vi "Populate Font Control.vi"(8 "error in (no error)":errorcluster, 10 "Font in":string, 11 "DNL_Font":refnum<vi>) -> (0 "error out":errorcluster, 2 "Font out":string)   [LabVIEW 2012]
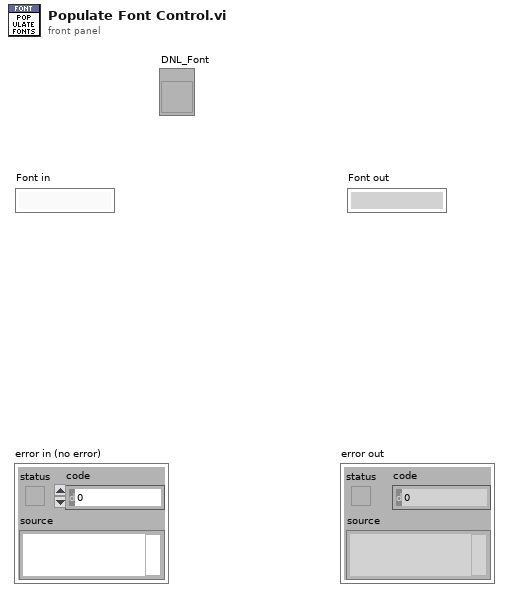
[diagram p1: front panel]
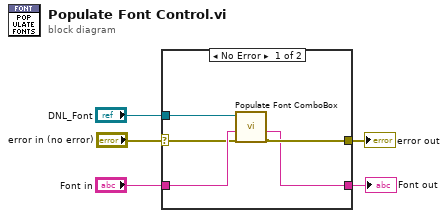
[diagram p0: block diagram]
diagram:
  n1 = case shown="No Error" "error in (no error)" {
    selector: "error in (no error)" -> [w7 w12]
    tunnel: [w9 w12] -> w4
    tunnel: "Font in" -> [w10 w11]
    tunnel: [w8 w11] -> w2
    tunnel: "DNL_Font" -> [w6 _]
    frame No Error {
      n2 = call <resource>:"Populate Font ComboBox.vi"("error in"=w7, "Font in"=w10, "CmbBox Refnum"=w6) -> ("error out"=w9:errorcluster, "Font out"=w8:string)  [unwired: 7 out]
    }
    frame Error {
    }
  }
  "error out" <- w4
  "Font out" <- w2
